vi "loadSettingsFromPath.vi"(8 "error in (no error)":errorcluster, 10 "Path":path, 11 "ICSettingsViewer in":refnum<class "ICSettingsViewer.lvclass">) -> (0 "error out":errorcluster, 3 "ICSettingsViewer out":refnum<class "ICSettingsViewer.lvclass">)   [LabVIEW 2011, in "Views.lvlib" / "Camera.lvlib" / "ICSettingsViewer.lvclass"]
uses:
  ICSettingsViewer.lvclass
  Tools/SettingsEventManager/SettingsEventsManager.lvclass
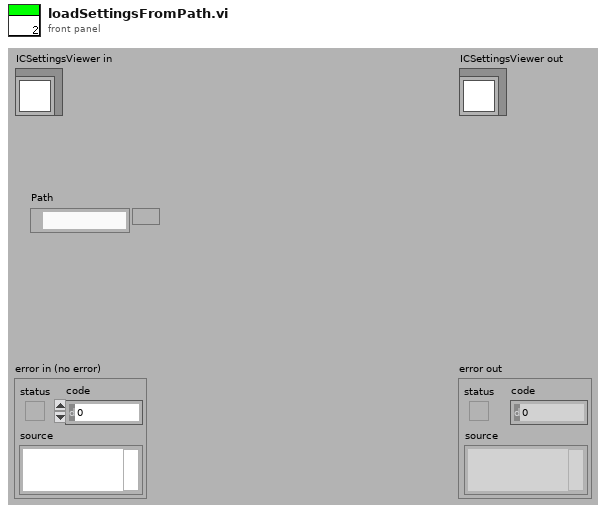
[diagram p1: front panel]
types:
  T1 = cluster{"settingsFrontEndEvents":cluster{"loadSettingsFromPath":refnum<user-event>, "lookUpElementEvent":refnum<user-event>, "saveSettings":refnum<user-event>, "loadSettings":refnum<user-event>, "close":refnum<user-event>, "replaceElement":refnum<user-event>, "findParentNodes":refnum<user-event>, "createNode":refnum<user-event>}, "settingBackEndEvents":cluster{"defaultSettingsPathRequest":refnum<user-event>, "searchResultEvent":refnum<user-event>, "settingsSaved":refnum<user-event>, "settingsLoaded":refnum<user-event>, "foundParentNode":refnum<user-event>}}
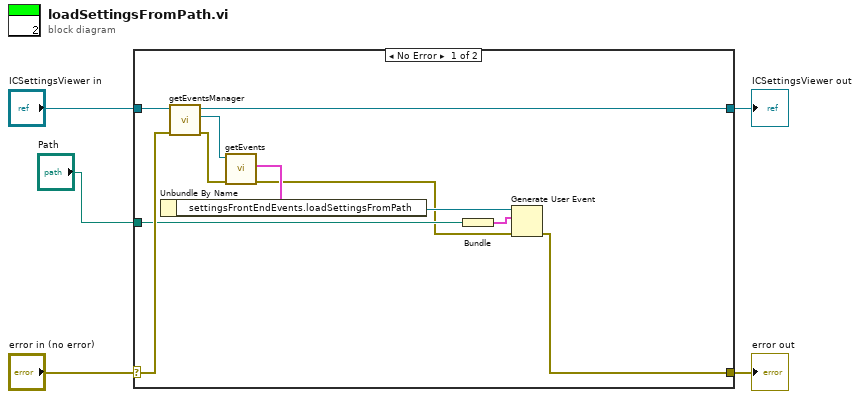
[diagram p0: block diagram]
diagram:
  n1 = case shown="No Error" "error in (no error)" {
    selector: "error in (no error)" -> [w13 w18]
    tunnel: [w6 w18] -> w4
    tunnel: [w15 w17] -> w2
    tunnel: "ICSettingsViewer in" -> [w16 w17]
    tunnel: "Path" -> [w9 _]
    frame No Error {
      n2 = call-dynamic "getEventsManager.vi"("error in (no error)"=w13, "SettingsViewer.lvclass in"=w16) -> ("error out"=w12:errorcluster, "Tools.lvlib:Settings.lvlib:SettingsEventsManager.lvclass"=w14:refnum<class "SettingsEventsManager.lvclass">, "SettingsViewer.lvclass out"=w15:refnum<class "ICSettingsViewer.lvclass">)  [unwired: 7 in]
      n3 = call-dynamic "getEvents.vi"("error in (no error)"=w12, "SettingsEventsManager in"=w14) -> ("error out"=w7:errorcluster, "settingsEvents"=w11:T1)  [unwired: 7 in, 1 out]
      n4 = Unbundle By Name(w11) -> ("settingsFrontEndEvents.loadSettingsFromPath"=w10:refnum<user-event>)
      n5 = Bundle("Path"=w9) -> (w8:cluster{"Path":path})  [unwired: 1 in]
      n6 = Generate User Event(user event=w10, event data cluster=w8, error in=w7) -> (error out=w6:errorcluster)  [unwired: 1 out]
    }
    frame Error {
    }
  }
  "error out" <- w4
  "ICSettingsViewer out" <- w2
